vi "告警触发机制 (子VI).vi"(9 "声光告警启用":bool, 10 "状态输出":bool, 11 "Digital输入":refnum<vi>) -> (2 "声光告警":bool, 3 "触发告警":bool)   [LabVIEW 2016, in "环境动力监测库.lvlib"]
uses:
  <vilib>/ptbypt/NI_PtbyPt.lvlib
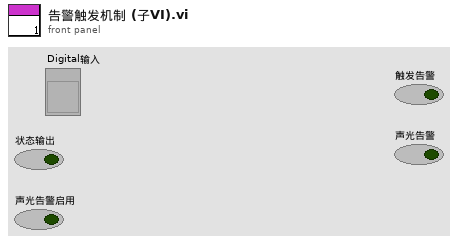
[diagram p1: front panel]
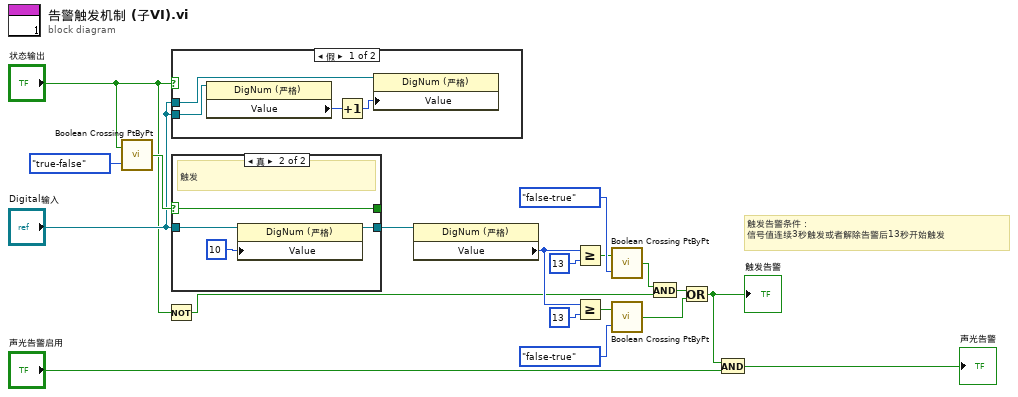
[diagram p0: block diagram]
diagram:
  # "触发告警条件：\n信号值连续3秒触发或者解除告警后13秒开始触发"
  n1 = call <vilib>:"Boolean Crossing PtByPt.vi"("direction"=enum16{"either", "false-true", "true-false"}."true-false", "input"="状态输出") -> ("crossing"=w12:bool)  [unwired: 1 in]
  n2 = Not(x="状态输出") -> (.not. x?=w4:bool)
  n3 = case shown="假" "状态输出" {
    tunnel: "Digital输入" -> [w21 _]
    tunnel: "Digital输入" -> [w20 _]
    frame False {
      n4 = property class="DigNum (严格)"(reference=w21) -> ("Value"=w22:u32)  [unwired: 1 in, 2 out]
      n5 = Increment(x=w22) -> (x+1=w23:u32)
      n6 = property class="DigNum (严格)"(reference=w20, "Value"=w23) -> ()  [unwired: 1 in, 2 out]
    }
    frame True {
    }
  }
  n7 = case shown="真" w12 {
    selector: w12 -> [w24 w26]
    tunnel: "Digital输入" -> [w25 w29]
    tunnel: [w25 w27] -> w11
    tunnel: [w24 w26] -> _
    frame False {
    }
    frame True {
      # "触发"
      n8 = property class="DigNum (严格)"(reference=w29, "Value"=u32 10 ("值")) -> (reference out=w27:refnum<vi>)  [unwired: 1 in, 1 out]
    }
  }
  n9 = property class="DigNum (严格)"(reference=w11) -> ("Value"=w7:u32)  [unwired: 1 in, 2 out]
  n10 = Greater Or Equal?(x=w7, y=u32 13) -> (x >= y?=w2:bool)
  n11 = Greater Or Equal?(x=w7, y=u32 13) -> (x >= y?=w17:bool)
  n12 = call <vilib>:"Boolean Crossing PtByPt.vi"("direction"=enum16{"either", "false-true", "true-false"}."false-true", "input"=w2) -> ("crossing"=w1:bool)  [unwired: 1 in]
  n13 = call <vilib>:"Boolean Crossing PtByPt.vi"("direction"=enum16{"either", "false-true", "true-false"}."false-true", "input"=w17) -> ("crossing"=w19:bool)  [unwired: 1 in]
  n14 = And(x=w1, y=w4) -> (x .and. y?=w6:bool)
  n15 = Or(x=w6, y=w19) -> (x .or. y?=w16:bool)
  "触发告警" <- w16
  n16 = And(x=w16, y="声光告警启用") -> (x .and. y?=→"声光告警":bool)
